vi "Spline Interpolation PtbyPt.vi"() -> ()   [LabVIEW 2023]
doc: "This example shows how to use point-by-point analysis to implement spline interpolation. The VI interpolates the values between the current point and the last point, at the position of <b>Ratio</b>*(current point - last point) + last point. <b>Ratio</b> must be in the range of [0, 1]. <b>Buffer length</b> is the length of each set of points."
uses:
  <vilib>/ptbypt/NI_PtbyPt.lvlib
panel:
  in  "Signal Input":u16(ring)=1 items=["sine", "square", "triangle", "sawtooth"]
  in  "Reinitialize":bool
  in  "Buffer length":i32(slide)=5 scale=2.0..20.0
  in  "Ratio":dbl(slide)=0.4 min=0.0 max=1.0 step=0.01 scale=0.0..1.0
  in  "Stop":bool
  out "Interpolation":cluster{dbl[], dbl[]}[](graph)
  # "Description: This VI shows how to use point-by-point analysis to implement spline interpolation.\nRequirements: LabVIEW Full Development System\nInstructions:\n1. Run the VI.\n2. Select the type of Signal Input and change the Ratio. Verify that the Spline will place an interpolation point between two consecutive samples.\n3. Click Stop to stop the VI."
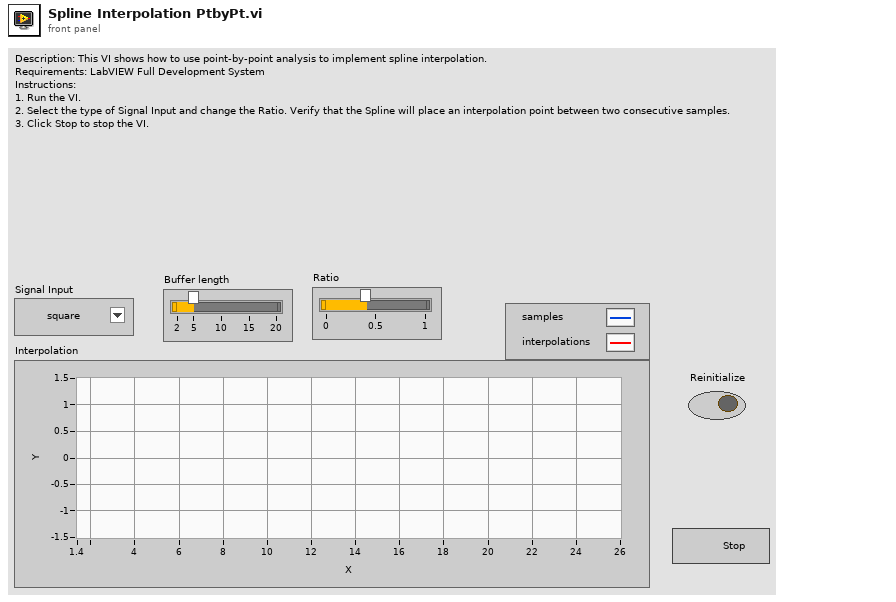
[diagram p1: front panel]
types:
  T1 = cluster{"Current Queue":dbl[], "Current Queue":dbl[]}
  T2 = cluster{"Current Queue":dbl[], "Current Queue":dbl[]}[]
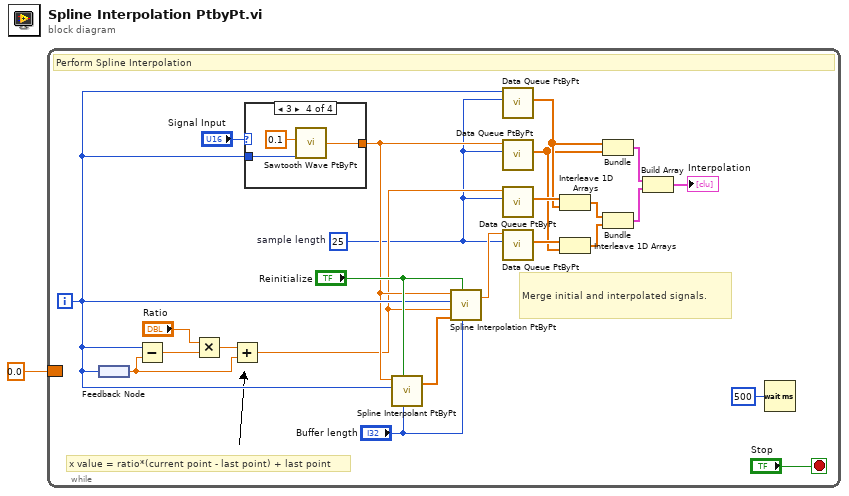
[diagram p0: block diagram]
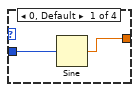
[diagram p2: hidden frame]
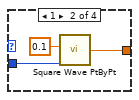
[diagram p3: hidden frame]
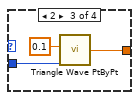
[diagram p4: hidden frame]
diagram:
  n1 = while {
    border: 0.0 -> [_]
    i -> [w13]
    stop <- "Stop" stop-if-true
    w8 = 25  # sample length
    # "Merge initial and interpolated signals."
    # "x value = ratio*(current point - last point) + last point"
    # "Perform Spline Interpolation"
    n2 = feedback-in #1(w13) -> ()
    n3 = feedback #1() -> (w22:dbl)
    n4 = Subtract(x=w13, y=w22) -> (x-y=w21:dbl)
    n5 = Multiply(x="Ratio", y=w21) -> (x*y=w20:dbl)
    n6 = Add(x=w20, y=w22) -> (x+y=w11:dbl)
    n7 = case shown="3" "Signal Input" {
      tunnel: w13 -> [w27 w29 w32 w35]
      tunnel: [w26 w28 w31 w34] -> w12
      frame 0, Default {
        n8 = Sine(x=w27) -> (sin(x)=w26:dbl)
      }
      frame 1 {
        n9 = call <vilib>:"Square Wave PtByPt.vi"("frequency"=0.1, "time"=w29) -> ("square wave"=w28:dbl)  [unwired: 3 in]
      }
      frame 2 {
        n10 = call <vilib>:"Triangle Wave PtByPt.vi"("time"=w32, "frequency"=0.1) -> ("triangle wave"=w31:dbl)  [unwired: 2 in]
      }
      frame 3 {
        n11 = call <vilib>:"Sawtooth Wave PtByPt.vi"("time"=w35, "frequency"=0.1) -> ("sawtooth wave"=w34:dbl)  [unwired: 2 in]
      }
    }
    n12 = call <vilib>:"Spline Interpolant PtByPt.vi"("sample length"="Buffer length", "initialize"="Reinitialize", "x"=w13, "y"=w12) -> ("Interpolant"=w16:dbl[])  [unwired: 2 in, 1 out]
    n13 = call <vilib>:"Spline Interpolation PtByPt.vi"("sample length"="Buffer length", "initialize"="Reinitialize", "Interpolant"=w16, "x value"=w11, "x"=w13, "y"=w12) -> ("interpolation value"=w9:dbl)  [unwired: 1 out]
    n14 = call <vilib>:"Data Queue PtByPt.vi"("sample length"=w8, "input data point"=w13) -> ("Current Queue"=w5:dbl[])  [unwired: 5 in, 4 out]
    n15 = call <vilib>:"Data Queue PtByPt.vi"("sample length"=w8, "input data point"=w12) -> ("Current Queue"=w3:dbl[])  [unwired: 5 in, 4 out]
    n16 = call <vilib>:"Data Queue PtByPt.vi"("sample length"=w8, "input data point"=w11) -> ("Current Queue"=w10:dbl[])  [unwired: 5 in, 4 out]
    n17 = call <vilib>:"Data Queue PtByPt.vi"("sample length"=w8, "input data point"=w9) -> ("Current Queue"=w4:dbl[])  [unwired: 5 in, 4 out]
    n18 = Interleave 1D Arrays(w10, w5) -> (w6:dbl[])
    n19 = Interleave 1D Arrays(w4, w3) -> (w2:dbl[])
    n20 = Bundle("Current Queue"=w5, "Current Queue"=w3) -> (w17:T1)  [unwired: 1 in]
    n21 = Bundle(w6, w2) -> (w23:cluster{dbl[], dbl[]})  [unwired: 1 in]
    n22 = Build Array(w17, w23) -> (→"Interpolation":T2)
    n23 = Wait (ms)(milliseconds to wait=u32 500) -> ()  [unwired: 1 out]
  }
